vi "Weibull Moments.vi"(9 "b":dbl=3.0, 10 "a":dbl=1.0) -> (0 "error":i32, 2 "variance":dbl=1.0, 3 "mean":dbl)   [LabVIEW 2017, in "NI_Gmath.lvlib"]
doc: "Returns the expected mean and variance of the random variate X, where X describes the selected distribution type. You must manually select the polymorphic instance to use."
uses:
  NI_Gmath.lvlib
  st_error_code.ctl
panel:
  # "Weibull Moments"
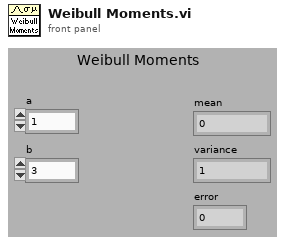
[diagram p1: front panel]
types:
  T1 = typedef "NI_Gmath.lvlib/st_error_code.ctl" = i32
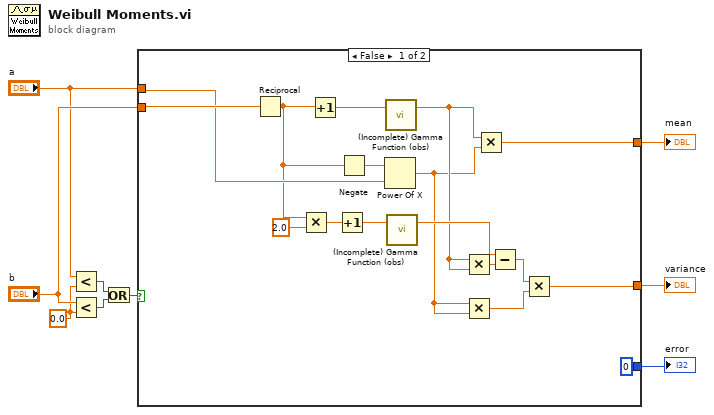
[diagram p0: block diagram]
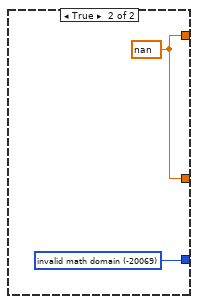
[diagram p2: hidden frame]
diagram:
  w6 = 0.0 ("y")
  n1 = Less?(x="a", y=w6) -> (x < y?=w2:bool)
  n2 = Less?(x="b", y=w6) -> (x < y?=w3:bool)
  n3 = Or(x=w2, y=w3) -> (x .or. y?=w4:bool)
  n4 = case shown="False" w4 {
    tunnel: "b" -> [w25 _]
    tunnel: [0 ("invalid math domain") w27] -> w9
    tunnel: [w21 w28] -> w8
    tunnel: "a" -> [w23 _]
    tunnel: [w10 w28] -> w1
    frame False {
      n5 = Reciprocal(x=w25) -> (1/x=w20:dbl)
      n6 = Multiply(x=w20, y=2.0) -> (x*y=w18:dbl)
      n7 = Increment(x=w20) -> (x+1=w24:dbl)
      n8 = Increment(x=w18) -> (x+1=w17:dbl)
      n9 = Negate(x=w20) -> (-x=w22:dbl)
      n10 = Power Of X(1:w23, 2:w22) -> (0:w13:dbl)
      n11 = call "(Incomplete) Gamma Function (obs).vi"("x"=w24) -> ("g(x, a)"=w14:dbl)  [unwired: 2 in]
      n12 = call "(Incomplete) Gamma Function (obs).vi"("x"=w17) -> ("g(x, a)"=w16:dbl)  [unwired: 2 in]
      n13 = Multiply(x=w14, y=w14) -> (x*y=w15:dbl)
      n14 = Multiply(x=w13, y=w13) -> (x*y=w11:dbl)
      n15 = Multiply(x=w14, y=w13) -> (x*y=w21:dbl)
      n16 = Subtract(x=w16, y=w15) -> (x-y=w12:dbl)
      n17 = Multiply(x=w12, y=w11) -> (x*y=w10:dbl)
    }
    frame True {
      w27 = T1 -20069 items=["invalid math domain"=-20069, "Fourier interpolation size m >= n"=-20070, "empty array"=-20003] ("stat interp error code")
      w28 = nan
    }
  }
  "mean" <- w8
  "error" <- w9
  "variance" <- w1
